vi "题目6.vi"() -> ()   [LabVIEW 2017]
panel:
  out "平均值":dbl
  out "最小值":dbl
  out "最大值":dbl
  out "波形图":cluster{dbl[]}[](graph)
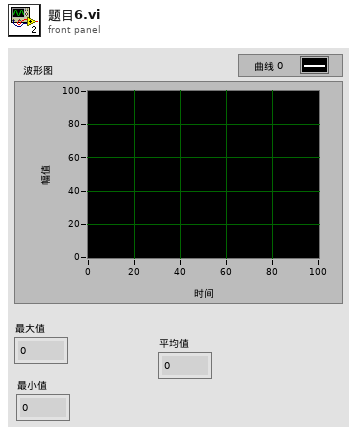
[diagram p1: front panel]
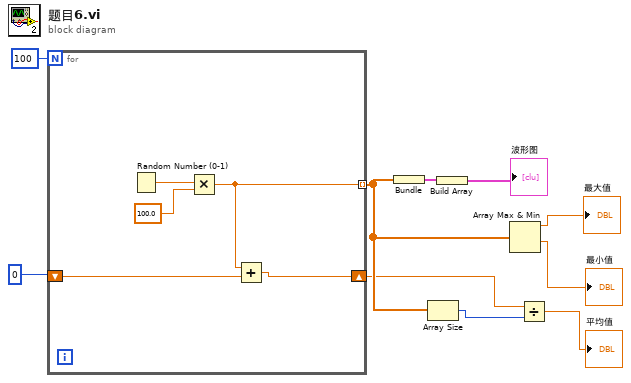
[diagram p0: block diagram]
diagram:
  n1 = for {
    N: 100 -> [_]
    tunnel: [w12] -> w5 mode=indexing
    shift-right: [w11] -> w2
    shift-left: 0 -> [w13]
    n2 = Random Number (0-1)() -> (number: 0 to 1=w15:dbl)
    n3 = Multiply(x=w15, y=100.0) -> (x*y=w12:dbl)
    n4 = Add(x=w12, y=w13) -> (x+y=w11:dbl)
  }
  n5 = Bundle(w5) -> (w9:cluster{dbl[]})  [unwired: 1 in]
  n6 = Array Size(array=w5) -> (size(s)=w4:i32)
  n7 = Build Array(w9) -> (→"波形图":cluster{dbl[]}[])
  n8 = Array Max & Min(array=w5) -> (max value=→"最大值":dbl, min value=→"最小值":dbl)  [unwired: 2 out]
  n9 = Divide(x=w2, y=w4) -> (x/y=→"平均值":dbl)
